vi "Initialise Termination Notifier.vi"(8 "error in (no error)":errorcluster) -> (0 "error out":errorcluster)   [LabVIEW 2017]
doc: "Initialise the termination notifier."
uses:
  Utilities/Application Globals.vi
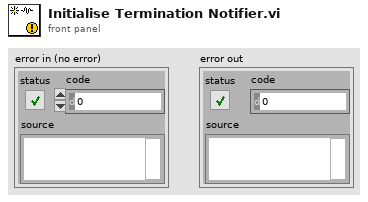
[diagram p1: front panel]
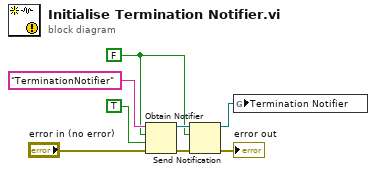
[diagram p0: block diagram]
diagram:
  w1 = FALSE ("notification")
  n1 = Obtain Notifier(name (unnamed)="TerminationNotifier", notification data type=w1, create if not found? (T)=TRUE, error in (no error)="error in (no error)") -> (notifier out=w5:refnum<notifier>, error out=w4:errorcluster)  [unwired: 1 out]
  n2 = Send Notification(notification=w1, notifier=w5, error in (no error)=w4) -> (notifier out=w6:refnum<notifier>, error out=→"error out":errorcluster)
  n3 = global write "Application Globals.vi" "Termination Notifier"(w6) -> ()
